vi "test_Host.vi"() -> ()   [LabVIEW 2015]
panel:
  in  "NS Smart":bool
  in  "NS Priority":bool
  in  "West Sensor":bool
  in  "East Sensor":bool
  in  "South Sensor":bool
  in  "North Sensor":bool
  out "Clock Frequency (Hz)":i16
  in  "PR1":bool
  in  "PR0":bool
  out "Time(s)":i16
  in  "Invert Physical Inputs?":bool
  out "EW RT button":bool
  out "NS RT button":bool
  out "EW phy button":bool
  out "NS phy button":bool
  out "EW Accepted":bool
  out "NS Accepted":bool
  in  "Accept Physical Inputs?":bool
  in  "NS Extend":bool
  in  "Stop":bool
  in  "Crosswalk(EW) new":bool
  in  "Crosswalk(NS) new":bool
  in  "Start":bool
  out "R(NS)":bool
  out "G(NS)":bool
  out "Y(NS)":bool
  out "R(EW)":bool
  out "G(EW)":bool
  out "Y(EW)":bool
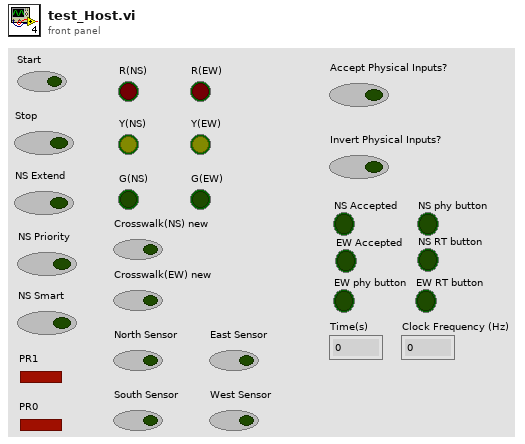
[diagram p1: front panel]
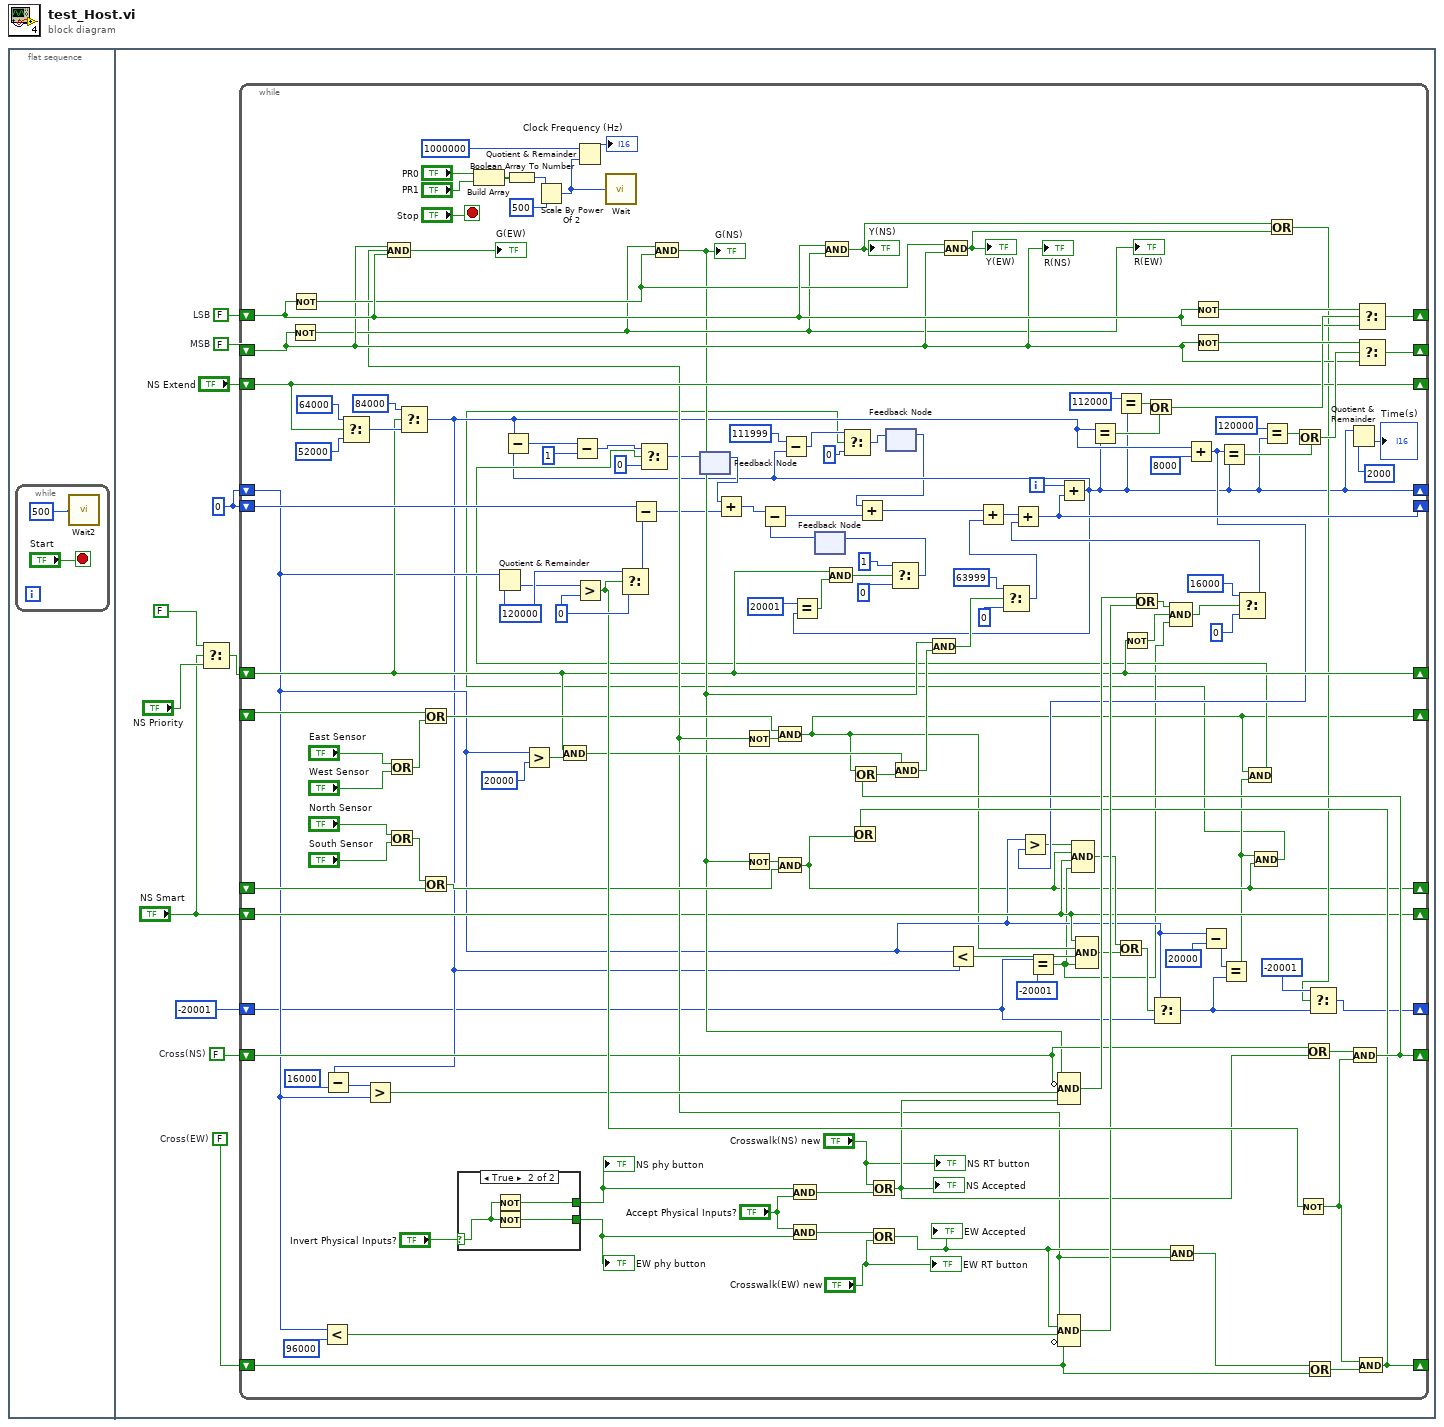
[diagram p0: block diagram]
diagram:
  n1 = flat-sequence {
    frame #0 {
      n2 = while {
        stop <- "Start" stop-if-true
        n3 = call "Wait2"("Count(mSec)"=u32 500) -> ()  [unwired: 1 out]
      }
    }
    frame #1 {
      w10 = FALSE  # Cross(NS)
      w11 = FALSE  # Cross(EW)
      w12 = FALSE  # MSB
      w13 = FALSE  # LSB
      w8 = 0
      n4 = Select(t=FALSE, s="NS Smart", f="NS Priority") -> (s? t:f=w6:bool)
      n5 = while {
        shift-right: [w21] -> _
        shift-left: w8 -> [w35]
        shift-right: [w72] -> _
        shift-left: w8 -> [w152]
        shift-right: [w149] -> _
        shift-left: w13 -> [w132]
        shift-right: [w148] -> _
        shift-left: w12 -> [w128]
        shift-right: [w59] -> _
        shift-left: w11 -> [w111]
        shift-right: [w64] -> _
        shift-left: w10 -> [w108]
        shift-right: [w129] -> _
        shift-left: "NS Extend" -> [w129]
        shift-right: [w61] -> _
        shift-left: w6 -> [w61]
        shift-right: [w29] -> _
        shift-left: _ -> [w90]
        shift-right: [w24] -> _
        shift-left: _ -> [w88]
        shift-right: [w36] -> _
        shift-left: "NS Smart" -> [w36]
        shift-right: [w48] -> _
        shift-left: -20001 -> [w31]
        i -> [w71]
        stop <- "Stop" stop-if-true
        w155 = 0
        w154 = 120000
        n6 = Not(x=w128) -> (.not. x?=w127:bool)
        "R(EW)" <- w127
        n7 = Not(x=w132) -> (.not. x?=w131:bool)
        n8 = Less?(x=w35, y=96000) -> (x < y?=w124:bool)
        n9 = Select(t=64000, s=w129, f=52000) -> (s? t:f=w93:i32)
        n10 = And(x=w128, y=w132) -> (x .and. y?=w65:bool)
        "G(EW)" <- w65
        n11 = Or(x="East Sensor", y="West Sensor") -> (x .or. y?=w91:bool)
        n12 = Or(x="North Sensor", y="South Sensor") -> (x .or. y?=w89:bool)
        n13 = Select(t=84000, s=w61, f=w93) -> (s? t:f=w32:i32)
        n14 = Subtract(x=w32, y=16000) -> (x-y=w110:i32)
        n15 = Greater?(x=w110, y=w35) -> (0:w126:bool)
        n16 = Or(x=w90, y=w91) -> (x .or. y?=w85:bool)
        n17 = Or(x=w89, y=w88) -> (x .or. y?=w84:bool)
        n18 = case shown="True" "Invert Physical Inputs?" {
          selector: "Invert Physical Inputs?" -> [w159 w160]
          tunnel: [w159 w162] -> w118
          tunnel: [w159 w161] -> w120
          frame False {
          }
          frame True {
            n19 = Not(x=w160) -> (.not. x?=w162:bool)
            n20 = Not(x=w160) -> (.not. x?=w161:bool)
          }
        }
        "NS phy button" <- w118
        "EW phy button" <- w120
        n21 = Build Array("PR0", "PR1") -> (w103:bool[])
        n22 = Quotient & Remainder(x=w35, y=w154) -> (floor(x/y)=w151:i32)  [unwired: 1 out]
        n23 = Boolean Array To Number(Boolean array=w103) -> (number=w102:u32)
        n24 = Greater?(x=w35, y=20000) -> (0:w80:bool)
        n25 = Scale By Power Of 2(n=w102, x=u32 500 ("Count(mSec)")) -> (x*2^n=w99:u32)
        n26 = And(x=w61, y=w80) -> (x .and. y?=w79:bool)
        n27 = Quotient & Remainder(x=1000000, y=w99) -> (floor(x/y)=→"Clock Frequency (Hz)":u32)  [unwired: 1 out]
        n28 = Greater?(x=w151, y=w155) -> (0:w150:bool)
        n29 = call "Wait"("Count(uSec)"=w99) -> ()  [unwired: 1 out]
        n30 = Select(t=w154, s=w150, f=w155) -> (s? t:f=w153:i32)
        n31 = Subtract(x=w152, y=w153) -> (x-y=w52:i32)
        n32 = And(x=w127, y=w131) -> (x .and. y?=w63:bool)
        "G(NS)" <- w63
        n33 = feedback #1() -> (w49:i32)  [unwired: 1 in]
        n34 = Add(x=w49, y=w52) -> (x+y=w53:i32)
        n35 = Not(x=w65) -> (.not. x?=w87:bool)
        n36 = Not(x=w63) -> (.not. x?=w86:bool)
        n37 = And(x=w85, y=w87) -> (x .and. y?=w29:bool)
        n38 = And(x=w86, y=w84) -> (x .and. y?=w24:bool)
        n39 = And(x=w118, y="Accept Physical Inputs?") -> (x .and. y?=w121:bool)
        n40 = And(x="Accept Physical Inputs?", y=w120) -> (x .and. y?=w116:bool)
        n41 = feedback #2() -> (w76:i32)  [unwired: 1 in]
        n42 = Subtract(x=w53, y=w76) -> (x-y=w18:i32)
        n43 = And(x=w132, y=w127) -> (x .and. y?=w42:bool)
        "Y(NS)" <- w42
        n44 = Or(x="Crosswalk(NS) new", y=w121) -> (x .or. y?=w109:bool)
        "NS Accepted" <- w109
        n45 = Or(x=w116, y="Crosswalk(EW) new") -> (x .or. y?=w112:bool)
        "EW Accepted" <- w112
        n46 = feedback #3() -> (w16:i32)  [unwired: 1 in]
        n47 = Add(x=w16, y=w18) -> (x+y=w15:i32)
        n48 = And(x=w131, y=w128) -> (x .and. y?=w41:bool)
        "Y(EW)" <- w41
        n49 = Less?(x=w35, y=w32) -> (x < y?=w57:bool)
        n50 = Equal?(x=w31, y=-20001) -> (x = y?=w26:bool)
        n51 = Compound Arithmetic op=AND(w63, invert w108, w126, w109) -> (w125:bool)
        n52 = Compound Arithmetic op=AND(w65, w112, w124, invert w111) -> (w123:bool)
        n53 = Compound Arithmetic op=AND(w36, w29, w57, w26) -> (w39:bool)
        n54 = Not(x=w61) -> (.not. x?=w27:bool)
        n55 = Or(x=w125, y=w123) -> (x .or. y?=w28:bool)
        n56 = And(x=w112, y=w65) -> (x .and. y?=w130:bool)
        n57 = Compound Arithmetic op=AND(w28, w27, w26) -> (w25:bool)
        n58 = Add(x=w32, y=8000) -> (x+y=w34:i32)
        n59 = Greater?(x=w35, y=w34) -> (0:w33:bool)
        n60 = Compound Arithmetic op=AND(w33, w24, w36, w26) -> (w37:bool)
        n61 = Or(x=w37, y=w39) -> (x .or. y?=w38:bool)
        n62 = Select(t=w35, s=w38, f=w31) -> (s? t:f=w55:i32)
        n63 = Not(x=w132) -> (.not. x?=w147:bool)
        n64 = Not(x=w128) -> (.not. x?=w146:bool)
        n65 = Subtract(x=w35, y=20000) -> (x-y=w46:i32)
        n66 = Equal?(x=w46, y=w55) -> (x = y?=w23:bool)
        n67 = Select(t=16000, s=w25, f=0) -> (s? t:f=w156:i32)
        n68 = And(x=w29, y=w23) -> (x .and. y?=w30:bool)
        n69 = And(x=w23, y=w24) -> (x .and. y?=w14:bool)
        n70 = Or(x=w42, y=w41) -> (x .or. y?=w40:bool)
        n71 = Not(x=w150) -> (.not. x?=w114:bool)
        n72 = Or(x=w108, y=w109) -> (x .or. y?=w113:bool)
        n73 = Or(x=w130, y=w111) -> (x .or. y?=w115:bool)
        n74 = Select(t=-20001, s=w40, f=w55) -> (s? t:f=w48:i32)
        n75 = And(x=w113, y=w114) -> (x .and. y?=w64:bool)
        n76 = Or(x=w29, y=w64) -> (x .or. y?=w56:bool)
        n77 = And(x=w79, y=w56) -> (x .and. y?=w67:bool)
        n78 = And(x=w63, y=w67) -> (x .and. y?=w66:bool)
        n79 = Select(t=63999, s=w66, f=0) -> (s? t:f=w73:i32)
        n80 = Add(x=w15, y=w73) -> (x+y=w75:i32)
        n81 = Add(x=w75, y=w156) -> (x+y=w72:i32)
        n82 = Add(x=w71, y=w72) -> (x+y=w21:i32)
        n83 = Subtract(x=w32, y=w21) -> (x-y=w45:i32)
        n84 = Subtract(x=w45, y=1) -> (x-y=w44:i32)
        n85 = Select(t=w44, s=w30, f=0) -> (s? t:f=w50:i32)
        n86 = feedback-in #1(w50) -> ()
        n87 = Subtract(x=111999, y=w21) -> (x-y=w19:i32)
        n88 = Equal?(x=20001, y=w21) -> (x = y?=w62:bool)
        n89 = And(x=w61, y=w62) -> (x .and. y?=w70:bool)
        n90 = Select(t=w19, s=w14, f=0) -> (s? t:f=w17:i32)
        n91 = feedback-in #3(w17) -> ()
        n92 = Select(t=1, s=w70, f=0) -> (s? t:f=w77:i32)
        n93 = feedback-in #2(w77) -> ()
        n94 = Equal?(x=w32, y=w21) -> (x = y?=w141:bool)
        n95 = Equal?(x=112000, y=w21) -> (x = y?=w142:bool)
        n96 = Or(x=w142, y=w141) -> (x .or. y?=w140:bool)
        n97 = Equal?(x=w34, y=w21) -> (x = y?=w138:bool)
        n98 = Equal?(x=120000, y=w21) -> (x = y?=w139:bool)
        n99 = Or(x=w139, y=w138) -> (x .or. y?=w135:bool)
        n100 = Quotient & Remainder(x=w21, y=2000) -> (floor(x/y)=→"Time(s)":i32)  [unwired: 1 out]
        n101 = And(x=w114, y=w115) -> (x .and. y?=w59:bool)
        n102 = Or(x=w24, y=w59) -> ()  [unwired: 1 out]
        n103 = Select(t=w147, s=w140, f=w132) -> (s? t:f=w149:bool)
        n104 = Select(t=w146, s=w135, f=w128) -> (s? t:f=w148:bool)
        "R(NS)" <- w128
        "NS RT button" <- "Crosswalk(NS) new"
        "EW RT button" <- "Crosswalk(EW) new"
      }
    }
  }
